vi "Explode String.vi"(5 "Remove Empty (F)":bool, 7 "Delimiter (,)":string=",", 11 "String":string) -> (3 "Array":string[](array[string]))   [LabVIEW 2020, in "Negentropic IDE.lvlib"]
uses:
  Negentropic IDE.lvlib
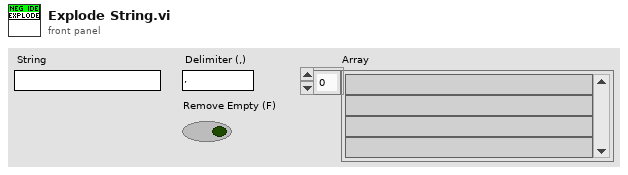
[diagram p1: front panel]
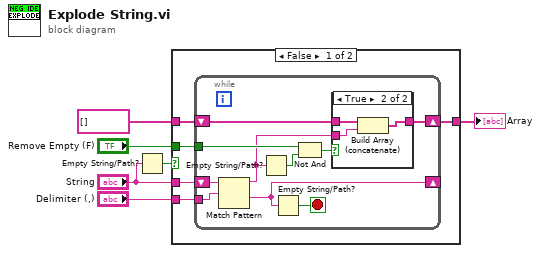
[diagram p0: block diagram]
diagram:
  n1 = Empty String/Path?(string/path="String") -> (empty?=w6:bool)
  n2 = case shown="False" w6 {
    tunnel: "String" -> [w9 _]
    tunnel: "Delimiter (,)" -> [w8 _]
    tunnel: "Remove Empty (F)" -> [w10 _]
    tunnel: string[] [] -> [w11 _]
    tunnel: [w7 _] -> w1
    frame False {
      n3 = while {
        shift-right: [w12] -> w7
        shift-left: w11 -> [w15]
        tunnel: w10 -> [w17]
        shift-right: [w19] -> _
        shift-left: w9 -> [w21]
        tunnel: w8 -> [w20]
        stop <- w18 stop-if-true
        n4 = Match Pattern(string=w21, regular expression=w20) -> (before substring=w13:string, after substring=w19:string)  [unwired: 1 in, 2 out]
        n5 = Empty String/Path?(string/path=w13) -> (empty?=w16:bool)
        n6 = Empty String/Path?(string/path=w19) -> (empty?=w18:bool)
        n7 = Not And(1:w16, 2:w17) -> (0:w14:bool)
        n8 = case shown="True" w14 {
          tunnel: w15 -> [w22 w25]
          tunnel: w13 -> [_ w24]
          tunnel: [w22 w23] -> w12
          frame False {
          }
          frame True {
            n9 = Build Array (concatenate)(w25, w24) -> (w23:string[])
          }
        }
      }
    }
    frame True {
    }
  }
  "Array" <- w1
